vi "Driver - DTACQ - Close TCP Connection.vi"(8 "error in":errorcluster, 11 "DTACQ Connection Data In":T1={"Description"="", "Address"="", "Port"=0, "timeout (ms)"=5000, "Termination Character"="\n", "TCP Connection Reference"=refnum, "Open Connection"=FALSE}) -> (0 "error out":errorcluster, 3 "DTACQ Connection Data Out":T1={"Description"="", "Address"="", "Port"=0, "timeout (ms)"=5000, "Termination Character"="\n", "TCP Connection Reference"=refnum, "Open Connection"=FALSE})   [LabVIEW 2017, in "Communications Library.lvlib"]
doc: "Closes a TCP connection to a DTACQ device.\n\nIf the connection is not marked as open, does nothing."
uses:
  Communications Library.lvlib
  Typedefs/DTACQ Connection Data--Cluster.ctl
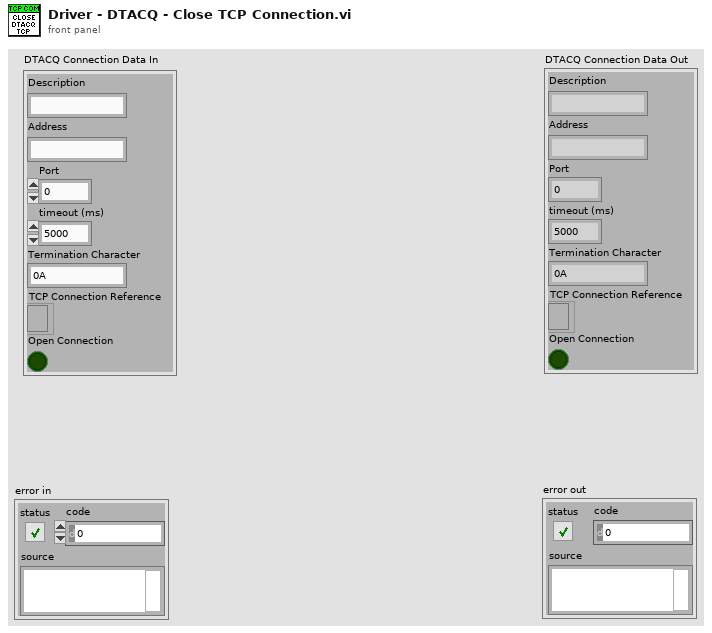
[diagram p1: front panel]
types:
  T1 = typedef "Communications Library.lvlib/DTACQ Connection Data--Cluster.ctl" = cluster{"Description":string, "Address":string, "Port":u16, "timeout (ms)":i32, "Termination Character":string, "TCP Connection Reference":refnum<k5>, "Open Connection":bool}
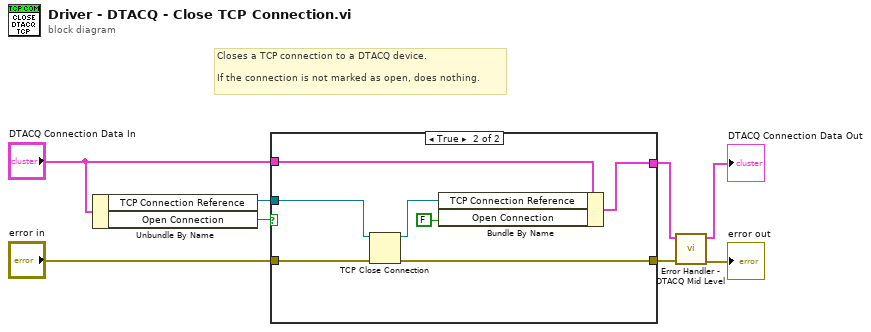
[diagram p0: block diagram]
diagram:
  # "Closes a TCP connection to a DTACQ device.\n\nIf the connection is not marked as open, does nothing."
  n1 = Unbundle By Name("DTACQ Connection Data In") -> ("TCP Connection Reference"=w5:refnum<k5>, "Open Connection"=w7:bool)
  n2 = case shown="True" w7 {
    tunnel: "error in" -> [w9 w16]
    tunnel: [w9 w15] -> w4
    tunnel: "DTACQ Connection Data In" -> [w10 w14]
    tunnel: [w10 w17] -> w3
    tunnel: w5 -> [_ w11]
    frame False {
    }
    frame True {
      n3 = TCP Close Connection(connection ID=w11, error in (no error)=w16) -> (connection ID out=w13:refnum<k5>, error out=w15:errorcluster)  [unwired: 1 in]
      n4 = Bundle By Name(cluster=w14, "TCP Connection Reference"=w13, "Open Connection"=FALSE) -> (w17:T1)
    }
  }
  n5 = call "Error Handler - DTACQ Mid Level.vi"("error in"=w4, "DTACQ Connection Data In"=w3) -> ("error out"=→"error out":errorcluster, "DTACQ Connection Data Out"=→"DTACQ Connection Data Out":T1)  [unwired: 7 in, 1 out]
